vi "frames.vi"() -> ()   [LabVIEW 2015]
panel:
  in  "DONE?":bool
  in  "Bending":bool[](array[boolean])=[FALSE, FALSE, FALSE, FALSE, FALSE, FALSE, FALSE, FALSE, FALSE, FALSE]
  out "Whole frame ID":string[](array[string])
  in  "?":string
  in  "?":string
  in  "?":string
  in  "?":string
  in  "?":string
  in  "?":string
  in  "?":string
  in  "?":string
  in  "?":string
  in  "Frame ID":string
  in  "?":i16(ring) items=["FRIM", "FDIM"]
  in  "?":i16(ring) items=["FRIM", "FDIM"]
  in  "?":i16(ring) items=["FRIM", "FDIM"]
  in  "?":i16(ring) items=["FRIM", "FDIM"]
  in  "?":i16(ring) items=["FRIM", "FDIM"]
  in  "?":i16(ring) items=["FRIM", "FDIM"]
  in  "?":i16(ring) items=["FRIM", "FDIM"]
  in  "?":i16(ring) items=["FRIM", "FDIM"]
  in  "?":i16(ring) items=["FRIM", "FDIM"]
  in  "Select frame type":i16(ring) items=["FRIM", "FDIM"]
  in  "Check Holes":bool[](array[boolean])=[FALSE, FALSE, FALSE, FALSE, FALSE, FALSE, FALSE, FALSE, FALSE, FALSE]
  out "Output file path":path
  in  "Thick_max":bool[](array[boolean])=[FALSE, FALSE, FALSE, FALSE, FALSE, FALSE, FALSE, FALSE, FALSE, FALSE]
  in  "Thick_min":bool[](array[boolean])=[FALSE, FALSE, FALSE, FALSE, FALSE, FALSE, FALSE, FALSE, FALSE, FALSE]
  in  "Wid_max":bool[](array[boolean])=[FALSE, FALSE, FALSE, FALSE, FALSE, FALSE, FALSE, FALSE, FALSE, FALSE]
  in  "Apri database":bool
  in  "Stop Button":bool
  in  "Refresh Button":bool
  in  "Crea file di testo":bool
  in  "Wid_min":bool[](array[boolean])=[FALSE, FALSE, FALSE, FALSE, FALSE, FALSE, FALSE, FALSE, FALSE, FALSE]
  # "Frame \"pass/no-pass\" tests"
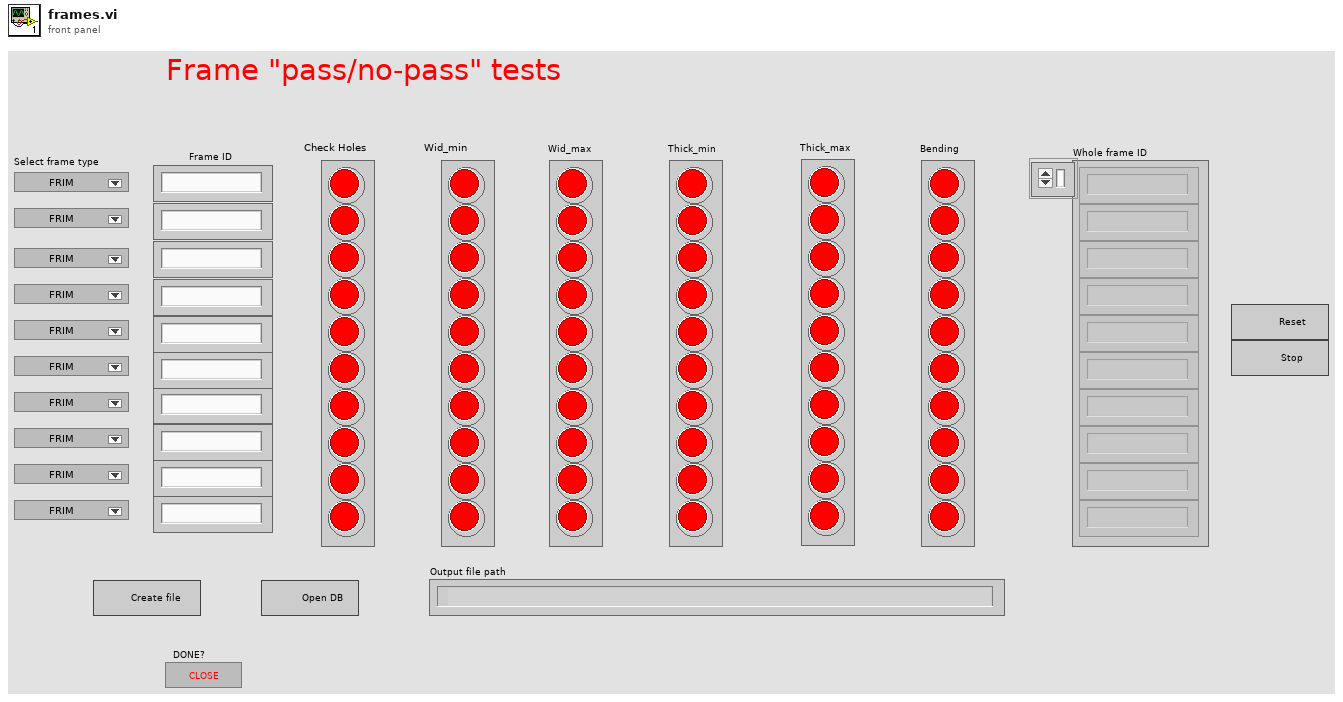
[diagram p1: front panel]
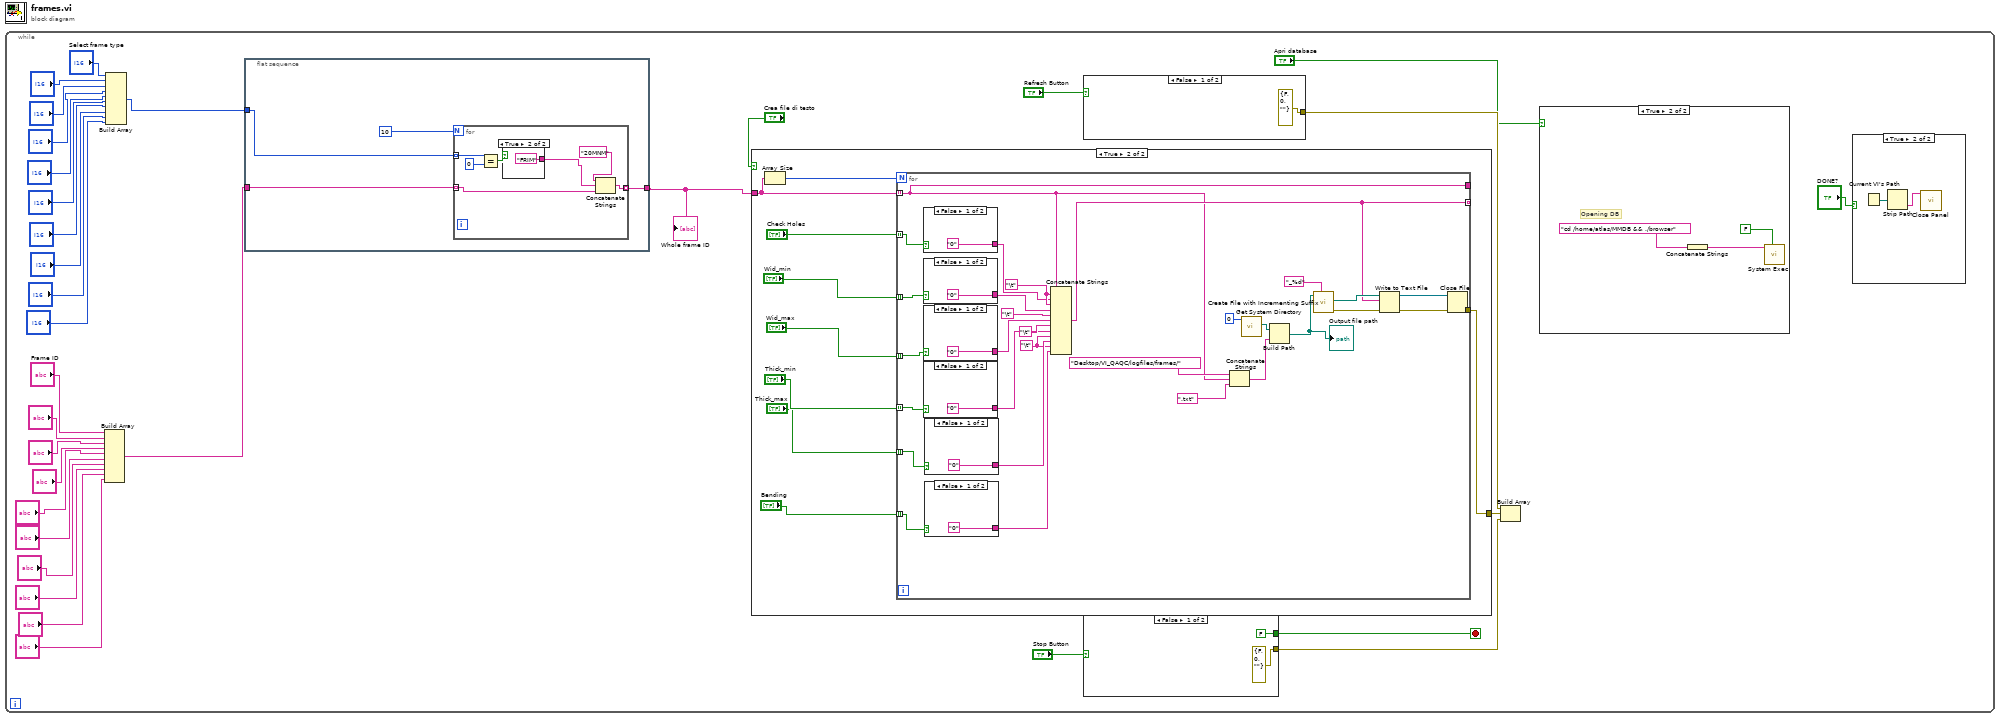
[diagram p0: block diagram]
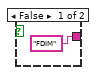
[diagram p3: hidden frame]
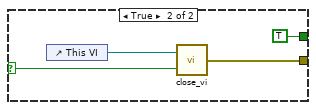
[diagram p5: hidden frame]
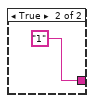
[diagram p7: hidden frame]
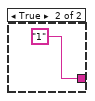
[diagram p8: hidden frame]
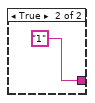
[diagram p9: hidden frame]
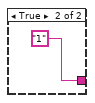
[diagram p10: hidden frame]
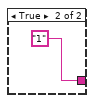
[diagram p11: hidden frame]
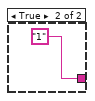
[diagram p12: hidden frame]
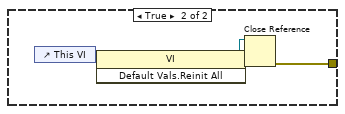
[diagram p13: hidden frame]
diagram:
  n1 = while {
    stop <- w26 stop-if-true
    n2 = Build Array("Frame ID", "?", "?", "?", "?", "?", "?", "?", "?", "?") -> (w7:string[])
    n3 = Build Array("Select frame type", "?", "?", "?", "?", "?", "?", "?", "?", "?") -> (w14:i16[])
    n4 = flat-sequence {
      tunnel: [w37] -> w30
      tunnel: w14 -> [w36]
      tunnel: w7 -> [w35]
      frame #0 {
        n5 = for {
          N: 10 -> [_]
          tunnel: [w45] -> w37 mode=indexing
          tunnel: w35 -> [w44] mode=indexing
          tunnel: w36 -> [w42] mode=indexing
          n6 = Equal?(x=w42, y=0) -> (x = y?=w40:bool)
          n7 = case shown="True" w40 {
            tunnel: ["FDIM" "FRIM"] -> w39
            frame False {
            }
            frame True {
            }
          }
          n8 = Concatenate Strings("20MNM", w39, w44) -> (w45:string)
        }
      }
    }
    n9 = case shown="True" "Crea file di testo" {
      tunnel: w30 -> [_ w64]
      tunnel: [_ w58] -> w6
      frame False {
      }
      frame True {
        n10 = Array Size(array=w64) -> (size(s)=w65:i32)
        n11 = for {
          N: w65 -> [_]
          tunnel: w64 -> [w71] mode=indexing
          tunnel: "Wid_min" -> [w95] mode=indexing
          tunnel: [w72] -> _ mode=indexing
          tunnel: [w71] -> _
          tunnel: "Wid_max" -> [w93] mode=indexing
          tunnel: "Thick_min" -> [w92] mode=indexing
          tunnel: "Thick_max" -> [w91] mode=indexing
          tunnel: "Check Holes" -> [w85] mode=indexing
          tunnel: [w69] -> w58
          tunnel: "Bending" -> [w68] mode=indexing
          w66 = "\t"
          w84 = "\t"
          n12 = case shown="False" w85 {
            tunnel: ["0" "1"] -> w83
            frame False {
            }
            frame True {
            }
          }
          n13 = case shown="False" w95 {
            tunnel: ["0" "1"] -> w94
            frame False {
            }
            frame True {
            }
          }
          n14 = case shown="False" w93 {
            tunnel: ["0" "1"] -> w89
            frame False {
            }
            frame True {
            }
          }
          n15 = case shown="False" w92 {
            tunnel: ["0" "1"] -> w87
            frame False {
            }
            frame True {
            }
          }
          n16 = case shown="False" w91 {
            tunnel: ["0" "1"] -> w86
            frame False {
            }
            frame True {
            }
          }
          n17 = case shown="False" w68 {
            tunnel: ["0" "1"] -> w67
            frame False {
            }
            frame True {
            }
          }
          n18 = Concatenate Strings(w71, w84, w83, w84, w94, "\t", w89, "\t", w87, w66, w86, w66, w67) -> (w72:string)
          n19 = Concatenate Strings("Desktop/VI_QAQC/logfiles/frames/", w71, ".txt") -> (w80:string)
          n20 = call <vilib>:"Get System Directory.vi"("system directory type"=0) -> ("system directory"=w79:path)  [unwired: 10 in]
          n21 = Build Path(base path=w79, name or relative path=w80) -> (appended path=w81:path)
          "Output file path" <- w81
          n22 = call <vilib>:"Create File with Incrementing Suffix.vi"("format string (\" (%d)\")"="_%d" ("format string (\" (%d)\")"), "file path"=w81) -> ("error out"=w73:errorcluster, "actual path"=w77:path)  [unwired: 7 in, 1 out]
          n23 = Write to Text File(file (use dialog)=w77, text=w72, error in=w73) -> (refnum out=w75:refnum<file>, error out=w74:errorcluster)  [unwired: 1 in, 1 out]
          n24 = Close File(refnum=w75, error in=w74) -> (error out=w69:errorcluster)  [unwired: 1 out]
        }
      }
    }
    n25 = case shown="False" "Refresh Button" {
      tunnel: [errorcluster {"status"=FALSE, "code"=0, "source"=""} ("error out") w109] -> w28
      frame False {
      }
      frame True {
        n26 = control-ref of="This VI"() -> (w112:refnum<vi>)
        n27 = invoke class="VI" method="Default Vals.Reinit All"(reference=w112) -> (reference out=w111:refnum<vi>, error out=w110:errorcluster)  [unwired: 2 in, 1 out]
        n28 = Close Reference(reference=w111, error in (no error)=w110) -> (error out=w109:errorcluster)
      }
    }
    n29 = case shown="False" "Stop Button" {
      selector: "Stop Button" -> [_ w55]
      tunnel: [errorcluster {"status"=FALSE, "code"=0, "source"=""} ("error out") w56] -> w29
      tunnel: [FALSE TRUE] -> w26
      frame False {
      }
      frame True {
        n30 = control-ref of="This VI"() -> (w53:refnum<vi>)
        n31 = call "close_vi.vi"("Process Stop Button"=w55, "reference"=w53) -> ("error out"=w56:errorcluster)
      }
    }
    n32 = Build Array(w28, w6, w29) -> ()  [unwired: 1 out]
    n33 = case shown="True" "Apri database" {
      frame False {
      }
      frame True {
        # "Opening DB"
        n34 = Concatenate Strings("cd /home/atlas/MMDB && ./browser") -> (w49:string)
        n35 = call <vilib>:"System Exec.vi"("wait until completion? (T)"=FALSE, "command line"=w49) -> ()  [unwired: 6 in, 4 out]
      }
    }
    n36 = case shown="True" "DONE?" {
      frame False {
      }
      frame True {
        n37 = Current VI's Path() -> (path=w33:path)
        n38 = Strip Path(path=w33) -> (name=w34:string)  [unwired: 1 out]
        n39 = call <vilib>:"Close Panel.vi"("VI name"=w34) -> ()  [unwired: 10 in, 1 out]
      }
    }
    "Whole frame ID" <- w30
  }
